vi "SongChosen.vi"(8 "error in (no error)":errorcluster, 10 "Click Details":T1, 11 "UI Refs":T2) -> (0 "error out":errorcluster)   [LabVIEW 2015]
uses:
  Controls & Type Defs/UI Data.ctl
  Controls & Type Defs/ClickDetails.ctl
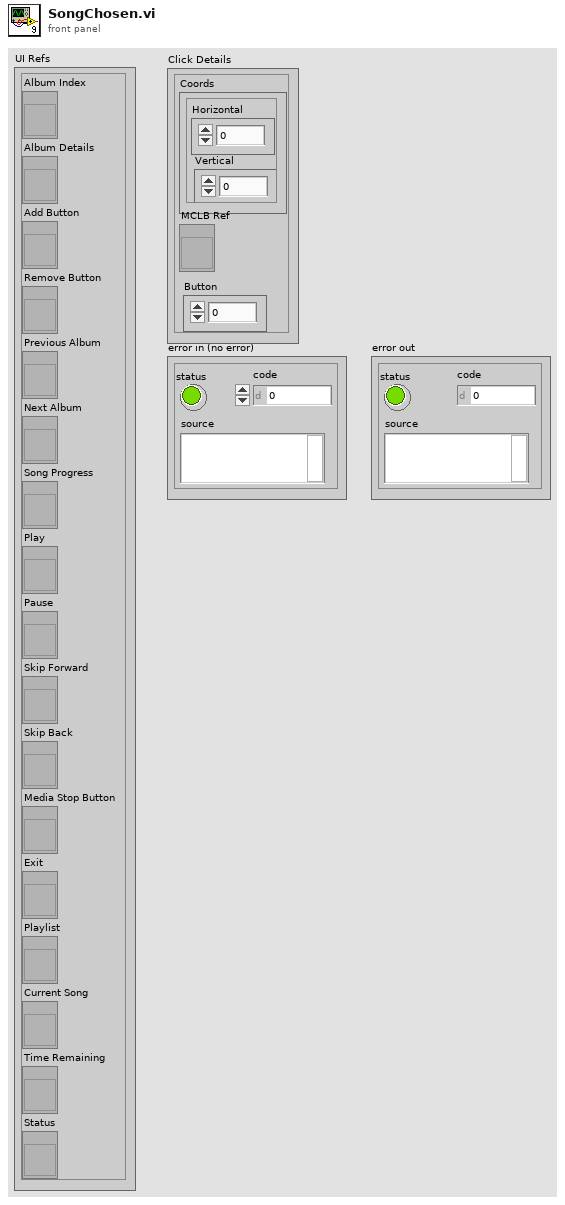
[diagram p1: front panel]
types:
  T1 = typedef "ClickDetails.ctl" = cluster{"Coords":cluster{"Vertical":i32, "Horizontal":i32}, "MCLB Ref":refnum<vi>, "Button":u16}
  T2 = typedef "UI Data.ctl" = cluster{"Album Index":refnum<vi>, "Album Details":refnum<vi>, "Add Button":refnum<vi>, "Remove Button":refnum<vi>, "Previous Album":refnum<vi>, "Next Album":refnum<vi>, "Song Progress":refnum<vi>, "Play":refnum<vi>, "Pause ":refnum<vi>, "Skip Forward":refnum<vi>, "Skip Back":refnum<vi>, "Media Stop Button":refnum<vi>, "Exit":refnum<vi>, "Playlist":refnum<vi>, "Current Song":refnum<vi>, "Time Remaining":refnum<vi>, "Status":refnum<vi>}
  T3 = typedef "LVRowAndColumnTypeDef.ctl" = cluster{"Row":i32, "Column":i32}
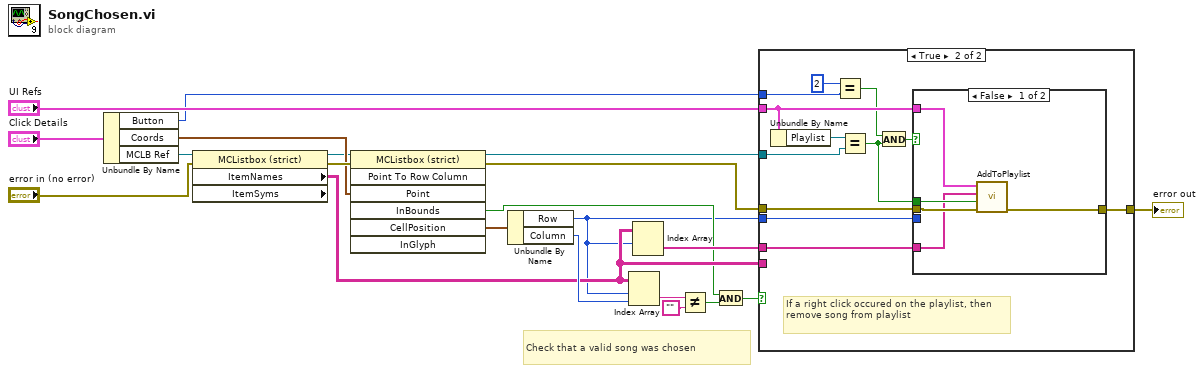
[diagram p0: block diagram]
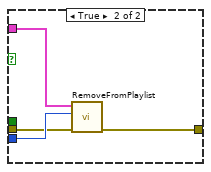
[diagram p3: hidden frame]
diagram:
  # "Check that a valid song was chosen"
  n1 = Unbundle By Name("Click Details") -> ("Button"=w2:u16, "Coords"=w20:cluster{"Vertical":i32, "Horizontal":i32}, "MCLB Ref"=w5:refnum<vi>)
  n2 = property class="MCListbox (strict)" props=["ItemNames", "ItemSyms"](reference=w5, error in="error in (no error)") -> (reference out=w4:refnum<vi>, error out=w21:errorcluster, "ItemNames"=w13:string[][])  [unwired: 1 out]
  n3 = invoke class="MCListbox (strict)" method="Point To Row Column"(reference=w4, error in=w21, "Point"=w20) -> (reference out=w3:refnum<vi>, error out=w14:errorcluster, "InBounds"=w9:bool, "CellPosition"=w17:T3)  [unwired: 4 in, 3 out]
  n4 = Unbundle By Name(w17) -> ("Row"=w1:i32, "Column"=w18:i32)
  n5 = Index Array(array=w13, index (row)=w1, index (col)=w18) -> (element=w16:string)
  n6 = Index Array(array=w13, index (row)=w1) -> (element=w12:string[])  [unwired: 1 in]
  n7 = Not Equal?(x=w16, y="") -> (x != y?=w8:bool)
  n8 = And(x=w9, y=w8) -> (x .and. y?=w7:bool)
  n9 = case shown="True" w7 {
    tunnel: "UI Refs" -> [_ w31]
    tunnel: w14 -> [w22 w34]
    tunnel: w13 -> [_ _]
    tunnel: w12 -> [_ w33]
    tunnel: [w22 w32] -> w11
    tunnel: w3 -> [_ w29]
    tunnel: w2 -> [_ w28]
    tunnel: w1 -> [_ w24]
    frame False {
    }
    frame True {
      # "If a right click occured on the playlist, then remove song from playlist"
      n10 = Unbundle By Name(w31) -> ("Playlist"=w30:refnum<vi>)
      n11 = Equal?(x=u16 2, y=w28) -> (x = y?=w25:bool)
      n12 = Equal?(x=w30, y=w29) -> (x = y?=w23:bool)
      n13 = And(x=w25, y=w23) -> (x .and. y?=w26:bool)
      n14 = case shown="False" w26 {
        tunnel: w31 -> [w39 w42]
        tunnel: w34 -> [w38 w40]
        tunnel: w33 -> [w35 _]
        tunnel: [w37 w41] -> w32
        tunnel: w24 -> [_ w43]
        tunnel: w23 -> [w36 _]
        frame False {
          n15 = call "AddToPlaylist.vi"("error in"=w38, "Playlist Clicked?"=w36, "NewSong"=w35, "UI Refs"=w39) -> ("error out"=w37:errorcluster)  [unwired: 7 in]
        }
        frame True {
          n16 = call "RemoveFromPlaylist.vi"("error in"=w40, "Song Index"=w43, "UI Refs"=w42) -> ("error out"=w41:errorcluster)  [unwired: 8 in]
        }
      }
    }
  }
  "error out" <- w11
